vi "ConvertDataDoubleToTaskStatus1.vi"(8 "error in (no error)":errorcluster, 9 "TaskStatus1":string(combo)="MaskValue", 10 "Double In":dbl[](array[numeric]), 11 "controller in":refnum<k24>) -> (0 "error out":errorcluster, 2 "TaskStatus1 Out":i32[](array[numeric]), 3 "controller out":refnum<k24>)   [LabVIEW 2010]
uses:
  c:/aerotech/controller/dev/A3200/pc/labview/2010/bin/Aerotech.A3200.dll
  bin/Aerotech.A3200.dll
  c:/aerotech/controller/dev/A3200/pc/labview/2010/bin/Aerotech.A3200.LabVIEW.dll
  bin/Aerotech.A3200.LabVIEW.dll
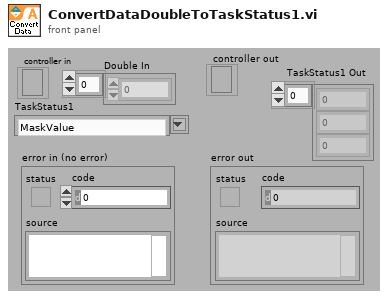
[diagram p1: front panel]
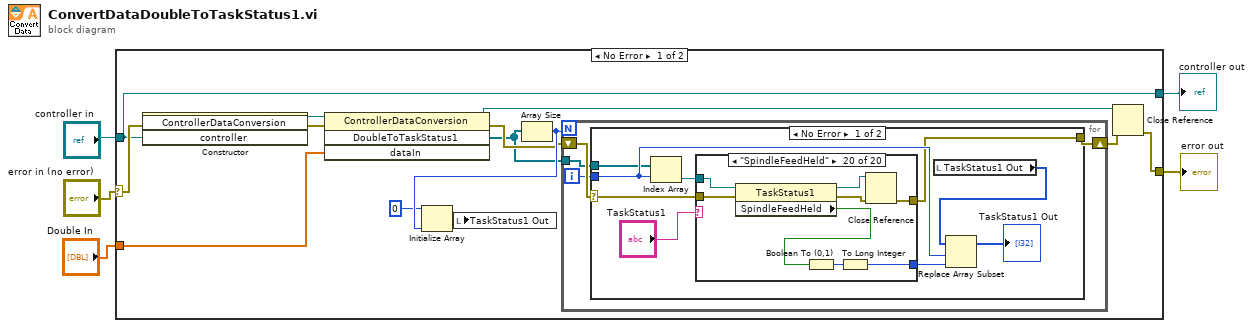
[diagram p0: block diagram]
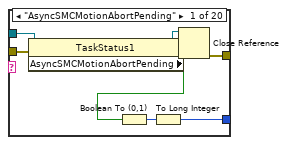
[diagram p2: hidden frame]
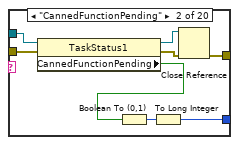
[diagram p3: hidden frame]
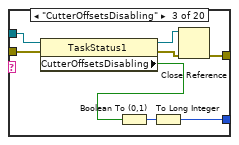
[diagram p4: hidden frame]
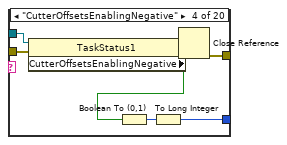
[diagram p5: hidden frame]
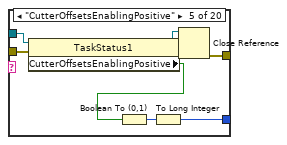
[diagram p6: hidden frame]
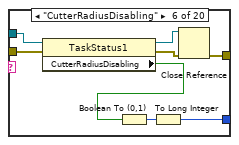
[diagram p7: hidden frame]
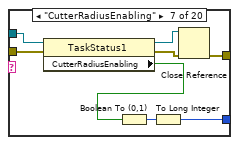
[diagram p8: hidden frame]
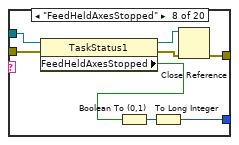
[diagram p9: hidden frame]
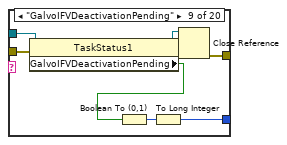
[diagram p10: hidden frame]
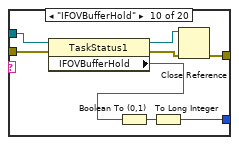
[diagram p11: hidden frame]
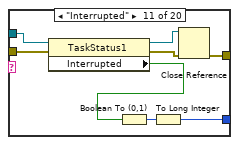
[diagram p12: hidden frame]
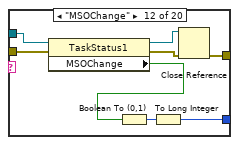
[diagram p13: hidden frame]
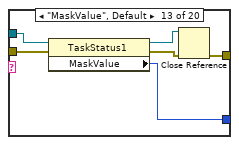
[diagram p14: hidden frame]
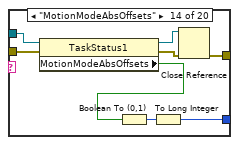
[diagram p15: hidden frame]
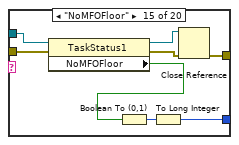
[diagram p16: hidden frame]
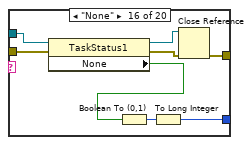
[diagram p17: hidden frame]
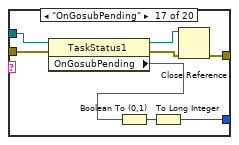
[diagram p18: hidden frame]
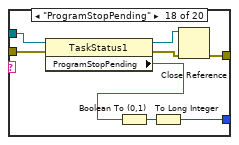
[diagram p19: hidden frame]
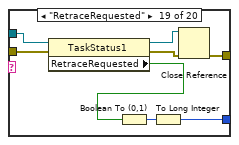
[diagram p20: hidden frame]
diagram:
  n1 = case shown="No Error" "error in (no error)" {
    selector: "error in (no error)" -> [w10 w192]
    tunnel: [w8 w192] -> w2
    tunnel: "controller in" -> [w7 w191]
    tunnel: "Double In" -> [w9 _]
    tunnel: [w7 w191] -> w1
    frame No Error {
      n2 = constructor class="ControllerDataConversion"(error in=w10, "controller"=w7) -> (reference out=w11:refnum<k24>, error out=w12:errorcluster)  [unwired: 2 in, 2 out]
      n3 = invoke class="ControllerDataConversion" method="DoubleToTaskStatus1"(reference=w11, error in=w12, "dataIn"=w9) -> (reference out=w13:refnum<k24>, error out=w15:errorcluster, "DoubleToTaskStatus1"=w14:refnum<k24>[])  [unwired: 1 in, 1 out]
      n4 = Array Size(array=w14) -> (size(s)=w18:i32)
      n5 = Initialize Array(0 ("element"), w18) -> (w6:i32[])
      n6 = local write "TaskStatus1 Out"(w6) -> ()
      n7 = for {
        N: w18 -> [_]
        tunnel: w14 -> [w20]
        shift-right: [w19] -> w16
        shift-left: w15 -> [w22]
        i -> [w21]
        n8 = case shown="No Error" w22 {
          selector: w22 -> [w26 w190]
          tunnel: [w23 w190] -> w19
          tunnel: w21 -> [w25 _]
          tunnel: w20 -> [w24 _]
          frame No Error {
            n9 = Index Array(array=w24, index=w25) -> (element=w31:refnum<k24>)
            n10 = case shown="\"SpindleFeedHeld\"" "TaskStatus1" {
              tunnel: w31 -> [w39 w47 w55 w63 w71 w79 w87 w95 w103 w111 w119 w127 w133 w141 w149 w157 w165 w173 w181 w189]
              tunnel: w26 -> [w36 w44 w52 w60 w68 w76 w84 w92 w100 w108 w116 w124 w130 w138 w146 w154 w162 w170 w178 w186]
              tunnel: [w34 w42 w50 w58 w66 w74 w82 w90 w98 w106 w114 w122 w128 w136 w144 w152 w160 w168 w176 w184] -> w29
              tunnel: [w33 w41 w49 w57 w65 w73 w81 w89 w97 w105 w113 w121 w129 w135 w143 w151 w159 w167 w175 w183] -> w23
              frame "AsyncSMCMotionAbortPending" {
                n11 = property class="TaskStatus1"(reference=w39, error in=w36) -> (reference out=w38:refnum<k24>, error out=w37:errorcluster, "AsyncSMCMotionAbortPending"=w32:bool)
                n12 = Boolean To (0,1)(Boolean=w32) -> (0, 1=w35:i16)
                n13 = To Long Integer(number=w35) -> (32bit integer=w34:i32)
                n14 = Close Reference(reference=w38, error in (no error)=w37) -> (error out=w33:errorcluster)
              }
              frame "CannedFunctionPending" {
                n15 = property class="TaskStatus1"(reference=w47, error in=w44) -> (reference out=w46:refnum<k24>, error out=w45:errorcluster, "CannedFunctionPending"=w40:bool)
                n16 = Boolean To (0,1)(Boolean=w40) -> (0, 1=w43:i16)
                n17 = To Long Integer(number=w43) -> (32bit integer=w42:i32)
                n18 = Close Reference(reference=w46, error in (no error)=w45) -> (error out=w41:errorcluster)
              }
              frame "CutterOffsetsDisabling" {
                n19 = property class="TaskStatus1"(reference=w55, error in=w52) -> (reference out=w54:refnum<k24>, error out=w53:errorcluster, "CutterOffsetsDisabling"=w48:bool)
                n20 = Boolean To (0,1)(Boolean=w48) -> (0, 1=w51:i16)
                n21 = To Long Integer(number=w51) -> (32bit integer=w50:i32)
                n22 = Close Reference(reference=w54, error in (no error)=w53) -> (error out=w49:errorcluster)
              }
              frame "CutterOffsetsEnablingNegative" {
                n23 = property class="TaskStatus1"(reference=w63, error in=w60) -> (reference out=w62:refnum<k24>, error out=w61:errorcluster, "CutterOffsetsEnablingNegative"=w56:bool)
                n24 = Boolean To (0,1)(Boolean=w56) -> (0, 1=w59:i16)
                n25 = To Long Integer(number=w59) -> (32bit integer=w58:i32)
                n26 = Close Reference(reference=w62, error in (no error)=w61) -> (error out=w57:errorcluster)
              }
              frame "CutterOffsetsEnablingPositive" {
                n27 = property class="TaskStatus1"(reference=w71, error in=w68) -> (reference out=w70:refnum<k24>, error out=w69:errorcluster, "CutterOffsetsEnablingPositive"=w64:bool)
                n28 = Boolean To (0,1)(Boolean=w64) -> (0, 1=w67:i16)
                n29 = To Long Integer(number=w67) -> (32bit integer=w66:i32)
                n30 = Close Reference(reference=w70, error in (no error)=w69) -> (error out=w65:errorcluster)
              }
              frame "CutterRadiusDisabling" {
                n31 = property class="TaskStatus1"(reference=w79, error in=w76) -> (reference out=w78:refnum<k24>, error out=w77:errorcluster, "CutterRadiusDisabling"=w72:bool)
                n32 = Boolean To (0,1)(Boolean=w72) -> (0, 1=w75:i16)
                n33 = To Long Integer(number=w75) -> (32bit integer=w74:i32)
                n34 = Close Reference(reference=w78, error in (no error)=w77) -> (error out=w73:errorcluster)
              }
              frame "CutterRadiusEnabling" {
                n35 = property class="TaskStatus1"(reference=w87, error in=w84) -> (reference out=w86:refnum<k24>, error out=w85:errorcluster, "CutterRadiusEnabling"=w80:bool)
                n36 = Boolean To (0,1)(Boolean=w80) -> (0, 1=w83:i16)
                n37 = To Long Integer(number=w83) -> (32bit integer=w82:i32)
                n38 = Close Reference(reference=w86, error in (no error)=w85) -> (error out=w81:errorcluster)
              }
              frame "FeedHeldAxesStopped" {
                n39 = property class="TaskStatus1"(reference=w95, error in=w92) -> (reference out=w94:refnum<k24>, error out=w93:errorcluster, "FeedHeldAxesStopped"=w88:bool)
                n40 = Boolean To (0,1)(Boolean=w88) -> (0, 1=w91:i16)
                n41 = To Long Integer(number=w91) -> (32bit integer=w90:i32)
                n42 = Close Reference(reference=w94, error in (no error)=w93) -> (error out=w89:errorcluster)
              }
              frame "GalvoIFVDeactivationPending" {
                n43 = property class="TaskStatus1"(reference=w103, error in=w100) -> (reference out=w102:refnum<k24>, error out=w101:errorcluster, "GalvoIFVDeactivationPending"=w96:bool)
                n44 = Boolean To (0,1)(Boolean=w96) -> (0, 1=w99:i16)
                n45 = To Long Integer(number=w99) -> (32bit integer=w98:i32)
                n46 = Close Reference(reference=w102, error in (no error)=w101) -> (error out=w97:errorcluster)
              }
              frame "IFOVBufferHold" {
                n47 = property class="TaskStatus1"(reference=w111, error in=w108) -> (reference out=w110:refnum<k24>, error out=w109:errorcluster, "IFOVBufferHold"=w104:bool)
                n48 = Boolean To (0,1)(Boolean=w104) -> (0, 1=w107:i16)
                n49 = To Long Integer(number=w107) -> (32bit integer=w106:i32)
                n50 = Close Reference(reference=w110, error in (no error)=w109) -> (error out=w105:errorcluster)
              }
              frame "Interrupted" {
                n51 = property class="TaskStatus1"(reference=w119, error in=w116) -> (reference out=w118:refnum<k24>, error out=w117:errorcluster, "Interrupted"=w112:bool)
                n52 = Boolean To (0,1)(Boolean=w112) -> (0, 1=w115:i16)
                n53 = To Long Integer(number=w115) -> (32bit integer=w114:i32)
                n54 = Close Reference(reference=w118, error in (no error)=w117) -> (error out=w113:errorcluster)
              }
              frame "MSOChange" {
                n55 = property class="TaskStatus1"(reference=w127, error in=w124) -> (reference out=w126:refnum<k24>, error out=w125:errorcluster, "MSOChange"=w120:bool)
                n56 = Boolean To (0,1)(Boolean=w120) -> (0, 1=w123:i16)
                n57 = To Long Integer(number=w123) -> (32bit integer=w122:i32)
                n58 = Close Reference(reference=w126, error in (no error)=w125) -> (error out=w121:errorcluster)
              }
              frame "MaskValue", Default {
                n59 = property class="TaskStatus1"(reference=w133, error in=w130) -> (reference out=w132:refnum<k24>, error out=w131:errorcluster, "MaskValue"=w128:i32)
                n60 = Close Reference(reference=w132, error in (no error)=w131) -> (error out=w129:errorcluster)
              }
              frame "MotionModeAbsOffsets" {
                n61 = property class="TaskStatus1"(reference=w141, error in=w138) -> (reference out=w140:refnum<k24>, error out=w139:errorcluster, "MotionModeAbsOffsets"=w134:bool)
                n62 = Boolean To (0,1)(Boolean=w134) -> (0, 1=w137:i16)
                n63 = To Long Integer(number=w137) -> (32bit integer=w136:i32)
                n64 = Close Reference(reference=w140, error in (no error)=w139) -> (error out=w135:errorcluster)
              }
              frame "NoMFOFloor" {
                n65 = property class="TaskStatus1"(reference=w149, error in=w146) -> (reference out=w148:refnum<k24>, error out=w147:errorcluster, "NoMFOFloor"=w142:bool)
                n66 = Boolean To (0,1)(Boolean=w142) -> (0, 1=w145:i16)
                n67 = To Long Integer(number=w145) -> (32bit integer=w144:i32)
                n68 = Close Reference(reference=w148, error in (no error)=w147) -> (error out=w143:errorcluster)
              }
              frame "None" {
                n69 = property class="TaskStatus1"(reference=w157, error in=w154) -> (reference out=w156:refnum<k24>, error out=w155:errorcluster, "None"=w150:bool)
                n70 = Boolean To (0,1)(Boolean=w150) -> (0, 1=w153:i16)
                n71 = To Long Integer(number=w153) -> (32bit integer=w152:i32)
                n72 = Close Reference(reference=w156, error in (no error)=w155) -> (error out=w151:errorcluster)
              }
              frame "OnGosubPending" {
                n73 = property class="TaskStatus1"(reference=w165, error in=w162) -> (reference out=w164:refnum<k24>, error out=w163:errorcluster, "OnGosubPending"=w158:bool)
                n74 = Boolean To (0,1)(Boolean=w158) -> (0, 1=w161:i16)
                n75 = To Long Integer(number=w161) -> (32bit integer=w160:i32)
                n76 = Close Reference(reference=w164, error in (no error)=w163) -> (error out=w159:errorcluster)
              }
              frame "ProgramStopPending" {
                n77 = property class="TaskStatus1"(reference=w173, error in=w170) -> (reference out=w172:refnum<k24>, error out=w171:errorcluster, "ProgramStopPending"=w166:bool)
                n78 = Boolean To (0,1)(Boolean=w166) -> (0, 1=w169:i16)
                n79 = To Long Integer(number=w169) -> (32bit integer=w168:i32)
                n80 = Close Reference(reference=w172, error in (no error)=w171) -> (error out=w167:errorcluster)
              }
              frame "RetraceRequested" {
                n81 = property class="TaskStatus1"(reference=w181, error in=w178) -> (reference out=w180:refnum<k24>, error out=w179:errorcluster, "RetraceRequested"=w174:bool)
                n82 = Boolean To (0,1)(Boolean=w174) -> (0, 1=w177:i16)
                n83 = To Long Integer(number=w177) -> (32bit integer=w176:i32)
                n84 = Close Reference(reference=w180, error in (no error)=w179) -> (error out=w175:errorcluster)
              }
              frame "SpindleFeedHeld" {
                n85 = property class="TaskStatus1"(reference=w189, error in=w186) -> (reference out=w188:refnum<k24>, error out=w187:errorcluster, "SpindleFeedHeld"=w182:bool)
                n86 = Boolean To (0,1)(Boolean=w182) -> (0, 1=w185:i16)
                n87 = To Long Integer(number=w185) -> (32bit integer=w184:i32)
                n88 = Close Reference(reference=w188, error in (no error)=w187) -> (error out=w183:errorcluster)
              }
            }
            n89 = local read "TaskStatus1 Out"() -> (w27:i32[])
            n90 = Replace Array Subset(array=w27, new element=w29, index=w25) -> (→"TaskStatus1 Out":i32[])
          }
          frame Error {
          }
        }
      }
      n91 = Close Reference(reference=w13, error in (no error)=w16) -> (error out=w8:errorcluster)
    }
    frame Error {
    }
  }
  "error out" <- w2
  "controller out" <- w1
